vi "Apply DSF Configuration.vi"(8 "error in (no error)":errorcluster, 10 "config path":path, 11 "Item Ref in":T1 format="%.0x") -> (0 "error out":errorcluster)   [LabVIEW 2017, in "DSF System Explorer.lvlib"]
uses:
  DSF System Explorer.lvlib
  <vilib>/NI Veristand/Custom Device API/Custom Device Item Ref.ctl
  DSF Core.lvlibp/Classes/Configuration/Configuration Session.lvclass
  <vilib>/NI Veristand/Custom Device API/Custom Device API.lvlib
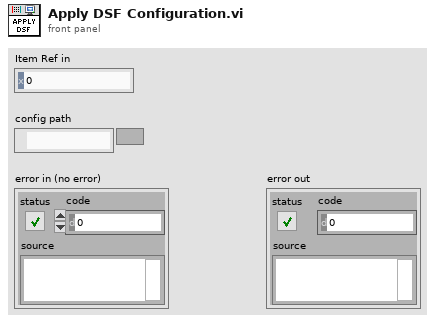
[diagram p1: front panel]
types:
  T1 = typedef "Custom Device API.lvlib/Custom Device Item Ref.ctl" = u64
  T2 = typedef "DSF Core.lvlibp/DSF Engine Framework Configuration.ctl" = cluster{"Plugins":T3[]}
  T3 = typedef "DSF Core.lvlibp/DSF Engine Plugin Configuration.ctl" = cluster{"name":string, "components":string[], "cycle timing":T4, "threads":T5[], "Transfer Groups":T7[], "settings":T6}
  T4 = typedef "DSF Core.lvlibp/DSF Timing Info.ctl" = cluster{"priority":u64, "decimation":u64, "offset":u64}
  T5 = typedef "DSF Core.lvlibp/DSF Engine Plugin Thread Configuration.ctl" = cluster{"buffer converter settings":T6, "transceiver settings":T6, "custom settings":T6, "processor":i32, "priority offset":i16}
  T6 = typedef "DSF Core.lvlibp/DSF Settings Info.ctl" = cluster{"key":string, "value":string}[]
  T7 = typedef "DSF Core.lvlibp/DSF Engine Transfer Group Configuration.ctl" = cluster{"name":string, "direction":T8, "cycle timing":T4, "thread index":i32, "settings":T6, "Transfers":T9[], "timeout behavior":T13}
  T8 = typedef "DSF Core.lvlibp/DSF Direction.ctl" = enum8{"Tx", "Rx"}
  T9 = typedef "DSF Core.lvlibp/DSF Engine Transfer Configuration.ctl" = cluster{"name":string, "byte order":T10, "settings":T6, "channels":T11[]}
  T10 = typedef "DSF Core.lvlibp/DSF Byte Order.ctl" = enum8{"big-endian", "little-endian"}
  T11 = typedef "DSF Core.lvlibp/DSF Engine Channel Configuration.ctl" = cluster{"string offset":u64, "string data type":T12, "engine data type":T12, "name":string, "settings":T6, "units":string}
  T12 = typedef "DSF Core.lvlibp/DSF Data Type.ctl" = enum8{"Bool", "SGL", "DBL", "I8", "I16", "I32", "I64", "U8", "U16", "U32", "U64"}
  T13 = typedef "DSF Core.lvlibp/DSF Timeout Behavior.ctl" = enum8{"Increment Late Count", "Throw Error"}
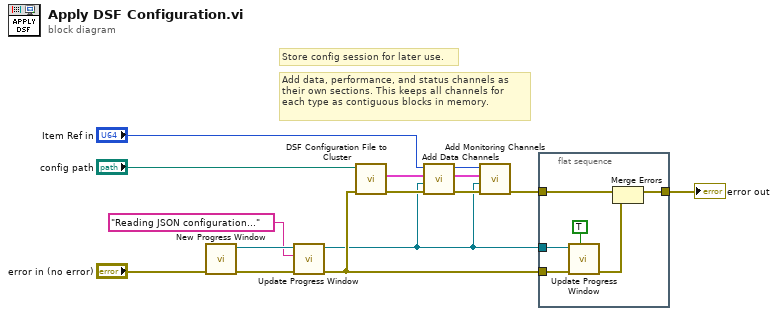
[diagram p0: block diagram]
diagram:
  # "Store config session for later use."
  # "Add data, performance, and status channels as their own sections. This keeps all channels for each type as contiguous blocks in memory."
  n1 = call "New Progress Window.vi"("error in (no error)"="error in (no error)") -> ("error out"=w12:errorcluster, "progress queue"=w11:refnum<queue>)  [unwired: 9 in]
  n2 = call "Update Progress Window.vi"("error in (no error)"=w12, "message (\"\")"="Reading JSON configuration..." ("message"), "progress queue in"=w11) -> ("error out"=w5:errorcluster, "progress queue out"=w1:refnum<queue>)  [unwired: 7 in]
  n3 = call "DSF Configuration File to Cluster.vi"("error in (no error)"=w5, "dsf configuration file path"="config path") -> ("error out"=w4:errorcluster, "framework configuration"=w2:T2)  [unwired: 7 in, 1 out]
  n4 = call "Add Data Channels.vi"("error in (no error)"=w4, "progress queue"=w1, "framework configuration"=w2, "Item Ref in"="Item Ref in") -> ("error out"=w7:errorcluster, "Item Ref out"=w14:T1)  [unwired: 6 in]
  n5 = call "Add Monitoring Channels.vi"("error in (no error)"=w7, "progress queue"=w1, "framework configuration"=w2, "Item Ref in"=w14) -> ("error out"=w8:errorcluster)  [unwired: 6 in, 1 out]
  n6 = flat-sequence {
    tunnel: w8 -> [w20]
    tunnel: [w18] -> w13
    tunnel: w5 -> [w16]
    tunnel: w1 -> [w15]
    frame #0 {
      n7 = call "Update Progress Window.vi"("stop (F)"=TRUE, "error in (no error)"=w16, "progress queue in"=w15) -> ("error out"=w19:errorcluster)  [unwired: 7 in, 1 out]
      n8 = Merge Errors(w20, w19) -> (w18:errorcluster)
    }
  }
  "error out" <- w13
